vi "ID Generator.vi"(1 "ID in":i32[](array[numeric])) -> (0 "ID out":i32[](array[numeric]))   [LabVIEW 2020]
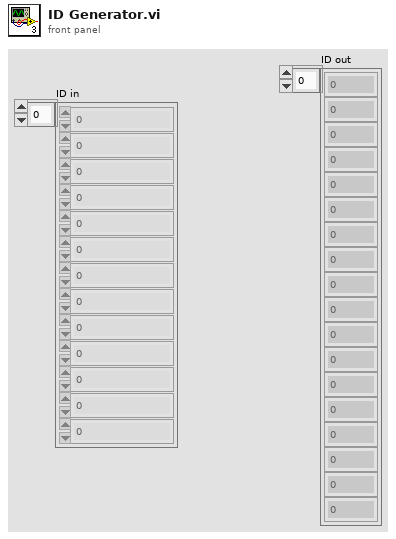
[diagram p1: front panel]
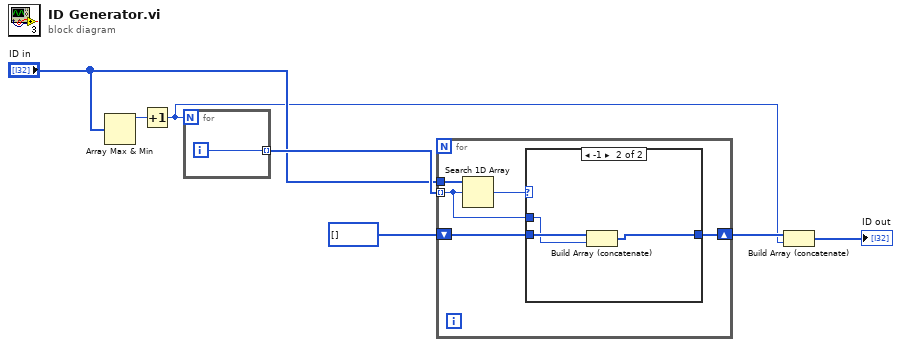
[diagram p0: block diagram]
diagram:
  n1 = Array Max & Min(array="ID in") -> (max value=w6:i32)  [unwired: 3 out]
  n2 = Increment(x=w6) -> (x+1=w1:i32)
  n3 = for {
    N: w1 -> [_]
    tunnel: [w8] -> w5 mode=indexing
    i -> [w8]
  }
  n4 = for {
    tunnel: "ID in" -> [w13]
    tunnel: w5 -> [w11] mode=indexing
    shift-right: [w9] -> w3
    shift-left: i32[] [] ("number") -> [w10]
    n5 = Search 1D Array(1D array=w13, element=w11) -> (index of element=w12:i32)  [unwired: 1 in]
    n6 = case shown="-1" w12 {
      tunnel: w11 -> [_ w16]
      tunnel: w10 -> [w14 w17]
      tunnel: [w14 w15] -> w9
      frame 0, Default {
      }
      frame -1 {
        n7 = Build Array (concatenate)(w17, w16) -> (w15:i32[])
      }
    }
  }
  n8 = Build Array (concatenate)(w3, w1) -> (→"ID out":i32[])
